vi "resultsColumnsCorrelations.vi"(10 "chValuesIn":string[](array[string]), 11 "chNamesIn":string[](array[string])) -> (2 "chValuesOut":string[](array[string]), 3 "chNamesOut":string[](array[string]))   [LabVIEW 2022 SP3]
uses:
  Globals/Meas_global.vi
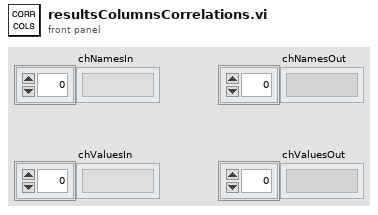
[diagram p1: front panel]
types:
  T1 = typedef "Analysis_info_cluster.ctl" = cluster{"Colour":u32, "Inst type":T2, "Inst name":string, "Symbol":string, "Code name":string, "Extra Info":string, "Inst Array":T3, "Extra Titles":string[], "Extra Values":string[], "U":dbl, "u^2":dbl, "u^3":dbl, "u^4":dbl, "Skew_u":dbl, "Kurt_u":dbl, "Sd Error in Mean":dbl, "% u'/U":dbl, "X":dbl, "Y":dbl, "Z":dbl, "Timescale integral Estimate":dbl, "Sd Error in Variance":dbl, "Calib File":path, "Calib Constants":dbl[], "Output Position":bool, "Stats":enum16{"None", "Basic", "Full"}, "Av Sampling Rate":dbl, "Av No of Samples":dbl, "Total Meas Time (s)":dbl, "ADAM Ch Name":string, "Max value":dbl, "Min value":dbl, "Req Sample Rate Hz":dbl, "Sync Delay Time (s)":dbl, "Ch No":i16, "Device":string, "Use Latest Calib":bool, "Port":string, "Metadata Ch Names":string[], "Metadata Ch Values":string[], "Label":string, "chState":T4}
  T2 = typedef "Inst_type.ctl" = enum16{"Raw voltage", "Raw with zero offsetting", "Propeller anemometer", "Pressure Transducer", "Pitot-static tube", "Hot wire", "Cross wire 1", "Cross wire 2", "Generic Linear", "Generic Polynomial", "Generic BackPoly", "Fast FID", "Thermocouple", "Cold wire", "Pulsed Wire", "LDA Vel", "LDA Tran time", "LDA Arr time", "Microphone"}
  T3 = typedef "Instrument_Array.ctl" = enum16{"PWA", "LDA", "Analogue"}
  T4 = typedef "channelState.ctl" = enum32{"No Selection", "Solo", "Mute"}
  T5 = typedef "Correlation_cluster1.ctl" = cluster{"U inst":string, "uw":dbl, "u^2w":dbl, "uw^2":dbl, "uw/u'w'":dbl, "W inst":string, "uw^3":dbl, "u^3w":dbl, "u^2w^2":dbl, "Index U":i32, "Index W":i32, "Error info":string[], "Paired Sampling Rate (Hz)":dbl, "u^2 Paired":dbl, "w^2 Paired":dbl, "Time Window (ms)":dbl}
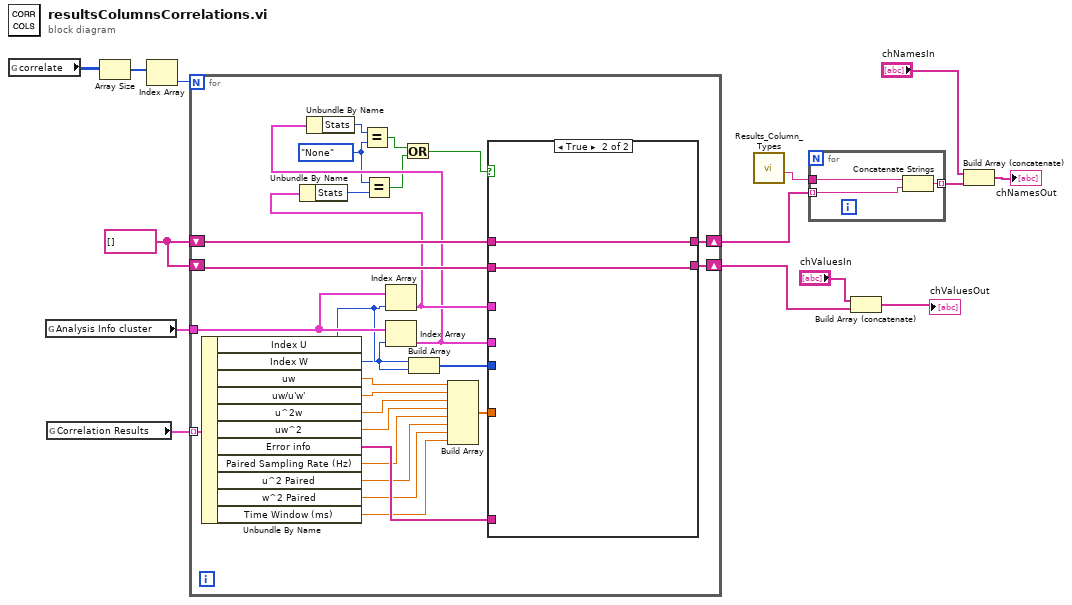
[diagram p0: block diagram]
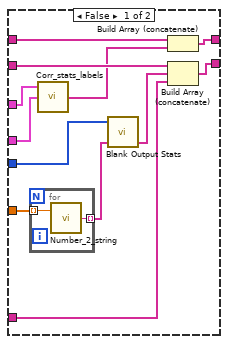
[diagram p2: hidden frame]
diagram:
  w7 = string[] []
  n1 = global read "Meas_global.vi" "correlate"() -> (w12:i32[][])
  n2 = global read "Meas_global.vi" "Analysis Info cluster"() -> (w14:T1[])
  n3 = global read "Meas_global.vi" "Correlation Results"() -> (w10:T5[])
  n4 = Array Size(array=w12) -> (size(s)=w11:i32[])
  n5 = Index Array(array=w11) -> (element=w13:i32)  [unwired: 1 in]
  n6 = for {
    N: w13 -> [_]
    shift-right: [w38] -> w9
    shift-left: w7 -> [w40]
    shift-right: [w41] -> w2
    shift-left: w7 -> [w39]
    tunnel: w10 -> [w37] mode=indexing
    tunnel: w14 -> [w36]
    w25 = enum16{"None", "Basic", "Full"}."None" ("Stats")
    n7 = Unbundle By Name(w37) -> ("Index U"=w17:i32, "Index W"=w16:i32, "uw"=w35:dbl, "uw/u'w'"=w34:dbl, "u^2w"=w33:dbl, "uw^2"=w32:dbl, "Error info"=w30:string[], "Paired Sampling Rate (Hz)"=w19:dbl, "u^2 Paired"=w21:dbl, "w^2 Paired"=w20:dbl, "Time Window (ms)"=w18:dbl)
    n8 = Index Array(array=w36, index=w17) -> (element=w29:T1)
    n9 = Unbundle By Name(w29) -> ("Stats"=w26:enum16{"None", "Basic", "Full"})
    n10 = Equal?(x=w25, y=w26) -> (x = y?=w23:bool)
    n11 = Index Array(array=w36, index=w16) -> (element=w28:T1)
    n12 = Unbundle By Name(w28) -> ("Stats"=w27:enum16{"None", "Basic", "Full"})
    n13 = Equal?(x=w27, y=w25) -> (x = y?=w24:bool)
    n14 = Or(x=w24, y=w23) -> (x .or. y?=w22:bool)
    n15 = Build Array(w17, w16) -> (w15:i32[])
    n16 = Build Array(w35, w34, w33, w32, w19, w21, w20, w18) -> (w31:dbl[])
    n17 = case shown="True" w22 {
      tunnel: [w53 w56] -> w41
      tunnel: w40 -> [w52 w57]
      tunnel: w39 -> [w51 w56]
      tunnel: [w50 w57] -> w38
      tunnel: w29 -> [w49 _]
      tunnel: w28 -> [w48 _]
      tunnel: w31 -> [w47 _]
      tunnel: w30 -> [w46 _]
      tunnel: w15 -> [w45 _]
      frame False {
        n18 = for {
          tunnel: w47 -> [w55] mode=indexing
          tunnel: [w54] -> w44 mode=indexing
          n19 = call "Number_2_string.vi"("number"=w55) -> ("String"=w54:string)  [unwired: 1 in]
        }
        n20 = call "Corr_stats_labels.vi"("Inst 2 Units"=w48, "Inst 1 Units"=w49) -> ("Output"=w42:string[])  [unwired: 1 in]
        n21 = call "Blank Output Stats.vi"("Ch Values in"=w44, "Indices"=w45) -> ("Ch Values Out"=w43:string[])  [unwired: 2 in, 1 out]
        n22 = Build Array (concatenate)(w52, w42) -> (w50:string[])
        n23 = Build Array (concatenate)(w51, w43, w46) -> (w53:string[])
      }
      frame True {
      }
    }
  }
  n24 = call "Results_Column_Types.vi"() -> ("Correlation"=w8:string)  [unwired: 9 in, 2 out]
  n25 = for {
    tunnel: w9 -> [w60] mode=indexing
    tunnel: [w59] -> w6 mode=indexing
    tunnel: w8 -> [w58]
    n26 = Concatenate Strings(w58, w60) -> (w59:string)
  }
  n27 = Build Array (concatenate)("chValuesIn", w2) -> (→"chValuesOut":string[])
  n28 = Build Array (concatenate)("chNamesIn", w6) -> (→"chNamesOut":string[])
